vi "UI.StimulusRestart.vi"(8 "error in (no error)":errorcluster, 11 "Cluster":T1={"NIVS.BaseLogPath"=path "", "NIVS.SystemDefinitionFile"=path "", "NIVS.Events"={"SequenceEvent"=refnum, "SystemChangeEvent"=refnum, "WorkspaceEvent"=refnum}, "NIVS.SequenceState"=enum."Idle", "NIVS.GatewayIPAddress"="", "NIVS.DataLogSpecRef"=refnum, "NIVS.DataLogManagerRef"=refnum, "NIVS.LogSessionGUID"="", "NIVS.WorkspaceManager"=refnum, "NIVS.Deployed"=FALSE, "NIVS.ProfileRef"=refnum, "NIVS.ProfileCallback"=refnum, "NIVS.SystemStateRefs"={"CustDatRef"=refnum, "EvtRef"=refnum}, "UI.Abort"=refnum, "UI.Pause"=refnum, "UI.EnableLogging"=refnum, "UI.Start"=refnum, "UI.LogChannels"=refnum, "UI.StartIteration"=refnum, "UI.StartStep"=refnum, "UI.Sequence"=refnum, "UI.PreviewMode"=refnum, "UI.Graph"=refnum, "UI.BaseFileName"=refnum, "UI.Profiles"=refnum, "UI.CurrentStep"=refnum, "UI.CurrentIteration"=refnum, "UI.TotalIterations"=refnum, "Sequence.AbortChannel"="", "Sequence.StepInfoChannel"="", "Sequence.Iterations"=0, "Sequence.IterationInfoChannel"="", "Sequence.#ofColumns"=0, "Events.State"=refnum, "Events.Test Result"=refnum, "Events.Progress"=refnum, "INI.Settings"={"Build Location"=path "C:/Simple Sequence Editor/SequenceRepo", "LoggingLocation"=path ""}, "UI.Skip"=refnum, "Sequence.SkipChannel"="", "Restart.Path"=path "", "UI.Duration"=refnum, "Sequence.DurationChannel"=""}) -> (0 "error out":errorcluster)   [LabVIEW 2013, in "Simple Sequence Tools - Execution.lvlib"]
uses:
  Simple Sequence Tools - Execution.lvlib
  Types/Main.StateVariables.ctl
  Types/Execute.UserEventRefs.ctl
  <vilib>/NI Veristand/Execution/Workspace/SystemStateRegEventRef.ctl
  Types/Execution.SequenceState.ctl
  <vilib>/NI Veristand/Execution/DataLogging/DataLoggingSpecification Ref.ctl
  NationalInstruments.VeriStand.ClientAPI
  <vilib>/NI Veristand/Execution/DataLogging/IDataLogging Ref.ctl
  <vilib>/NI Veristand/Execution/Workspace/WorkspaceAPI.ctl
  NationalInstruments.VeriStand.RealTimeSequenceDefinitionApi
  <vilib>/NI Veristand/Execution/Workspace/SystemStateEventRef.ctl
  Shared/Types/INI.Settings
  <vilib>/NI Veristand/Execution/Workspace/NI_VS Workspace ExecutionAPI.lvlib
  <vilib>/NI Veristand/Execution/DataLogging/NI_VS Data Logging API.lvlib
  Shared/Simple Sequence Tools - Shared.lvlib
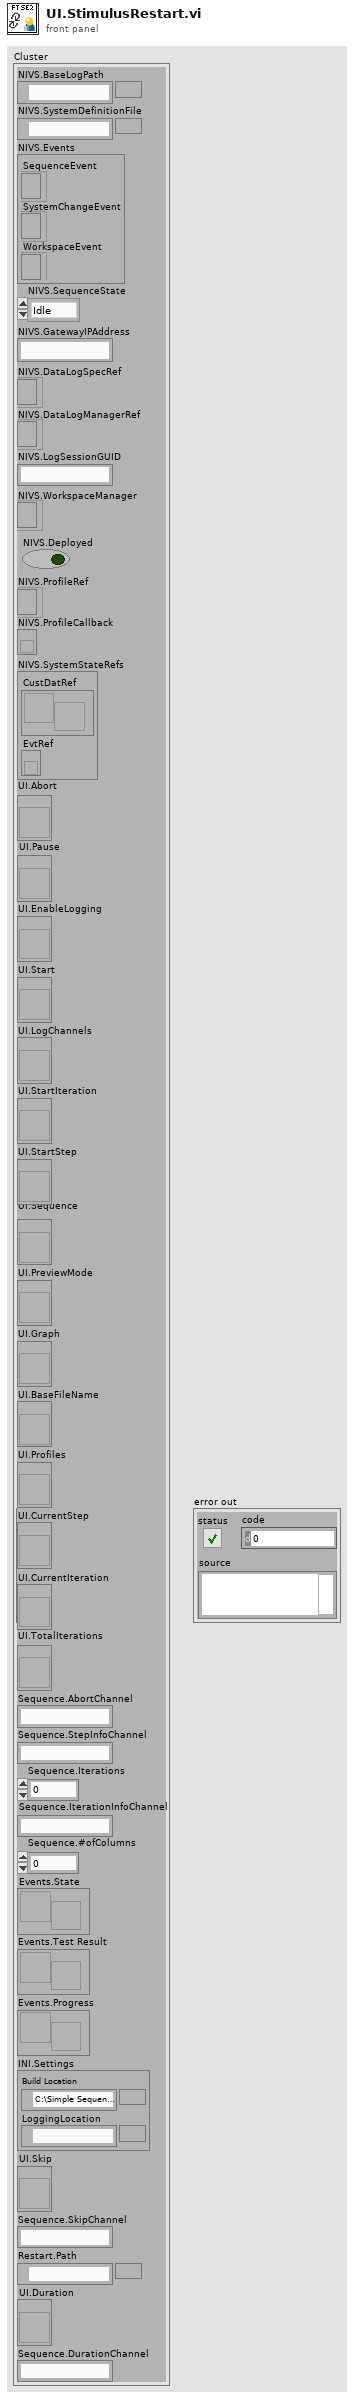
[diagram p1: front panel]
types:
  T1 = typedef "Simple Sequence Tools - Execution.lvlib/Main.StateVariables.ctl" = cluster{"NIVS.BaseLogPath":path, "NIVS.SystemDefinitionFile":path, "NIVS.Events":T2, "NIVS.SequenceState":T4, "NIVS.GatewayIPAddress":string, "NIVS.DataLogSpecRef":T5, "NIVS.DataLogManagerRef":T6, "NIVS.LogSessionGUID":string, "NIVS.WorkspaceManager":T7, "NIVS.Deployed":bool, "NIVS.ProfileRef":refnum<k24>, "NIVS.ProfileCallback":refnum<k27>, "NIVS.SystemStateRefs":T8, "UI.Abort":refnum<vi>, "UI.Pause":refnum<vi>, "UI.EnableLogging":refnum<vi>, "UI.Start":refnum<vi>, "UI.LogChannels":refnum<vi>, "UI.StartIteration":refnum<vi>, "UI.StartStep":refnum<vi>, "UI.Sequence":refnum<vi>, "UI.PreviewMode":refnum<vi>, "UI.Graph":refnum<vi>, "UI.BaseFileName":refnum<vi>, "UI.Profiles":refnum<vi>, "UI.CurrentStep":refnum<vi>, "UI.CurrentIteration":refnum<vi>, "UI.TotalIterations":refnum<vi>, "Sequence.AbortChannel":string, "Sequence.StepInfoChannel":string, "Sequence.Iterations":u32, "Sequence.IterationInfoChannel":string, "Sequence.#ofColumns":i32, "Events.State":refnum<user-event>, "Events.Test Result":refnum<user-event>, "Events.Progress":refnum<user-event>, "INI.Settings":T9, "UI.Skip":refnum<vi>, "Sequence.SkipChannel":string, "Restart.Path":path, "UI.Duration":refnum<vi>, "Sequence.DurationChannel":string}
  T2 = typedef "Simple Sequence Tools - Execution.lvlib/Execute.UserEventRefs.ctl" = cluster{"SequenceEvent":refnum<event-registration>, "SystemChangeEvent":T3, "WorkspaceEvent":refnum<event-registration>}
  T3 = typedef "NI_VS Workspace ExecutionAPI.lvlib/SystemStateRegEventRef.ctl" = refnum<event-registration>
  T4 = typedef "Simple Sequence Tools - Execution.lvlib/Execution.SequenceState.ctl" = enum16{"Idle", "Initializing", "Running", "Paused", "Finalizing", "Complete"}
  T5 = typedef "NI_VS Data Logging API.lvlib/DataLoggingSpecification Ref.ctl" = refnum<k24>
  T6 = typedef "NI_VS Data Logging API.lvlib/IDataLogging Ref.ctl" = refnum<k24>
  T7 = typedef "NI_VS Workspace ExecutionAPI.lvlib/WorkspaceAPI.ctl" = refnum<k24>
  T8 = typedef "NI_VS Workspace ExecutionAPI.lvlib/SystemStateEventRef.ctl" = cluster{"CustDatRef":refnum<user-event>, "EvtRef":refnum<k27>}
  T9 = typedef "Simple Sequence Tools - Shared.lvlib/INI.Settings" = cluster{"Build Location":path, "LoggingLocation":path}
  T10 = enum8{"Enabled", "Disabled", "Disabled and Grayed Out"}
  T11 = typedef "Simple Sequence Tools - Execution.lvlib/Restart.Settings" = cluster{"LogFile":path, "Log Settings":T12[], "StimulusProfile":path, "StopIteration":u32, "StopStep":u32, "Log Channels":T16, "Base File Name":string, "Enable Logging":bool, "Profile":string, "StopDuration":dbl}
  T12 = typedef "NI_VS Data Logging API.lvlib/TDMS Channel Group.ctl" = cluster{"Group Name":string, "Group Description":string, "Group Properties":T13[], "Channels":T14[], "Time Channel Options":T15, "Time Channel Name":string}
  T13 = typedef "NI_VS Data Logging API.lvlib/TDMS Property.ctl" = cluster{"Name":string, "Value":variant}
  T14 = typedef "NI_VS Data Logging API.lvlib/TDMS Channel.ctl" = cluster{"Channel Name":string, "Channel Path":string, "Channel Description":string, "Channel Properties":T13[]}
  T15 = typedef "NI_VS Data Logging API.lvlib/Time Channel Options.ctl" = enum16{"No Time Channel", "Absolute Time", "System Time", "System Time - Microseconds", "Absolute Time as Double"}
  T16 = typedef "Simple Sequence Tools - Execution.lvlib/Log.SelectedChannels.ctl" = enum16{"Channels (No System Channel)", "Aliases", "All"}
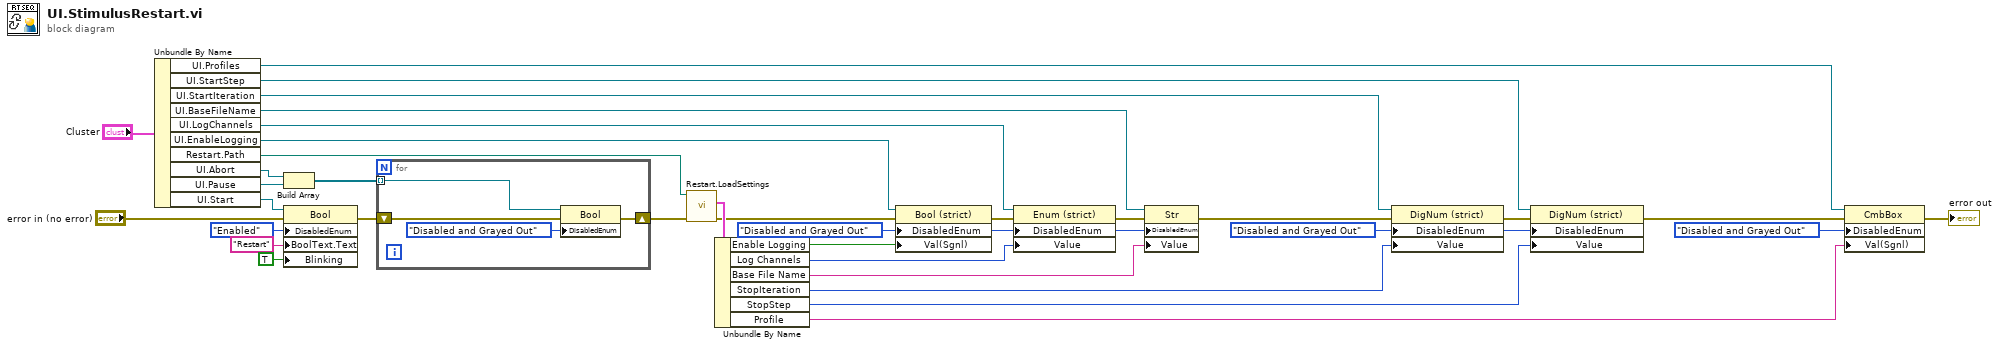
[diagram p0: block diagram]
diagram:
  w1 = T10."Disabled and Grayed Out" ("Disabled")
  w16 = T10."Disabled and Grayed Out" ("Disabled")
  n1 = Unbundle By Name("Cluster") -> ("UI.Profiles"=w35:refnum<vi>, "UI.StartStep"=w17:refnum<vi>, "UI.StartIteration"=w18:refnum<vi>, "UI.BaseFileName"=w23:refnum<vi>, "UI.LogChannels"=w33:refnum<vi>, "UI.EnableLogging"=w32:refnum<vi>, "Restart.Path"=w4:path, "UI.Abort"=w29:refnum<vi>, "UI.Pause"=w30:refnum<vi>, "UI.Start"=w24:refnum<vi>)
  n2 = Build Array(w29, w30) -> (w31:refnum<vi>[])
  n3 = property class="Bool"(reference=w24, error in="error in (no error)", "DisabledEnum"=T10."Enabled" ("Disabled"), "BoolText.Text"="Restart" ("Boolean Text.Text"), "Blinking"=TRUE) -> (error out=w25:errorcluster)  [unwired: 1 out]
  n4 = for {
    tunnel: w31 -> [w39] mode=indexing
    shift-right: [w37] -> w9
    shift-left: w25 -> [w36]
    n5 = property class="Bool"(reference=w39, error in=w36, "DisabledEnum"=T10."Disabled and Grayed Out" ("Disabled")) -> (error out=w37:errorcluster)  [unwired: 1 out]
  }
  n6 = call "Restart.LoadSettings.vi"("error in"=w9, "path (use dialog)"=w4) -> ("error out"=w8:errorcluster, "Restart Settings"=w15:T11)  [unwired: 7 in, 1 out]
  n7 = Unbundle By Name(w15) -> ("Enable Logging"=w7:bool, "Log Channels"=w6:T16, "Base File Name"=w5:string, "StopIteration"=w14:u32, "StopStep"=w13:u32, "Profile"=w3:string)
  n8 = property class="Bool (strict)"(reference=w32, error in=w8, "DisabledEnum"=w16, "Val(Sgnl)"=w7) -> (error out=w34:errorcluster)  [unwired: 1 out]
  n9 = property class="Enum (strict)"(reference=w33, error in=w34, "DisabledEnum"=w16, "Value"=w6) -> (error out=w22:errorcluster)  [unwired: 1 out]
  n10 = property class="Str"(reference=w23, error in=w22, "DisabledEnum"=w16, "Value"=w5) -> (error out=w10:errorcluster)  [unwired: 1 out]
  n11 = property class="DigNum (strict)"(reference=w18, error in=w10, "DisabledEnum"=w1, "Value"=w14) -> (error out=w20:errorcluster)  [unwired: 1 out]
  n12 = property class="DigNum (strict)"(reference=w17, error in=w20, "DisabledEnum"=w1, "Value"=w13) -> (error out=w19:errorcluster)  [unwired: 1 out]
  n13 = property class="CmbBox"(reference=w35, error in=w19, "DisabledEnum"=T10."Disabled and Grayed Out" ("Disabled"), "Val(Sgnl)"=w3) -> (error out=→"error out":errorcluster)  [unwired: 1 out]
